vi "Type Definition Name To Message Name.vi"(11 "type definition name":string="ni.protobuf.types.lvlib:ni_protobuf_types_DoubleXYData.ctl") -> (3 "message name":string)   [LabVIEW 2020, in "MeasurementLink Measurement Server.lvlib"]
uses:
  MeasurementLink Measurement Server.lvlib
  <vilib>/regexp/Match Regular Expression.xnode
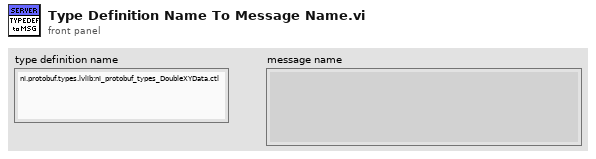
[diagram p1: front panel]
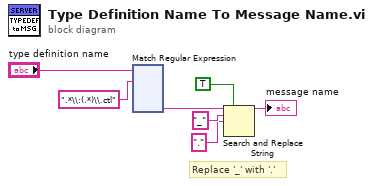
[diagram p0: block diagram]
diagram:
  # "Replace '_' with '.'"
  n1 = xnode "Match Regular Expression"("input string"="type definition name", "regular expression"=".*\\:(.*)\\.ctl") -> ("submatch 1"=w1:string)  [unwired: 4 in, 5 out]
  n2 = Search and Replace String(replace all?=TRUE ("replace all? (F)"), input string=w1, search string="_", replace string="." ("replace string (\"\")")) -> (result string=→"message name":string)  [unwired: 4 in, 3 out]
